vi "DB-通用exe查询模块.vi"(8 "error in (no error)":errorcluster, 9 "解析模式":enum16{"仅数值", "仅字符串", "数值与字符串", "不转换", "不抓取"}(ring)=enum."不抓取" caption="解析模式(不抓取)", 10 "SQL query":string, 11 "数据库连接引用":T1) -> (0 "error out":errorcluster, 1 "字符串数据":string[][](array[string]), 2 "数值数据":dbl[][](array[numeric]), 3 "数据库连接引用out":T1, 4 "recordset data":variant[][](array[variant]))   [LabVIEW 2017]
uses:
  <vilib>/addons/database/Connection.llb/Conn ObjectReference.ctl
  <vilib>/addons/database/Connection.llb/Conn Execute.vi
  <vilib>/addons/database/Recordset.llb/Rec Fetch Recordset Data (R).vi
  <vilib>/addons/database/Recordset.llb/Rec Destroy - Connection.vi
  <vilib>/addons/database/_DB Variant To Data/Database Variant To Data.xnode
  <vilib>/addons/database/NI_Database_API.lvlib
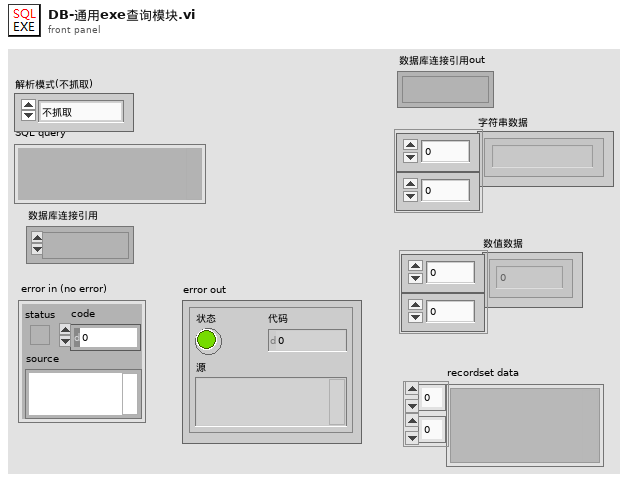
[diagram p1: front panel]
types:
  T1 = typedef "NI_Database_API.lvlib/Conn ObjectReference.ctl" = refnum<k1>
  T2 = typedef "NI_Database_API.lvlib/Rec ObjectReference.ctl" = refnum<k1>
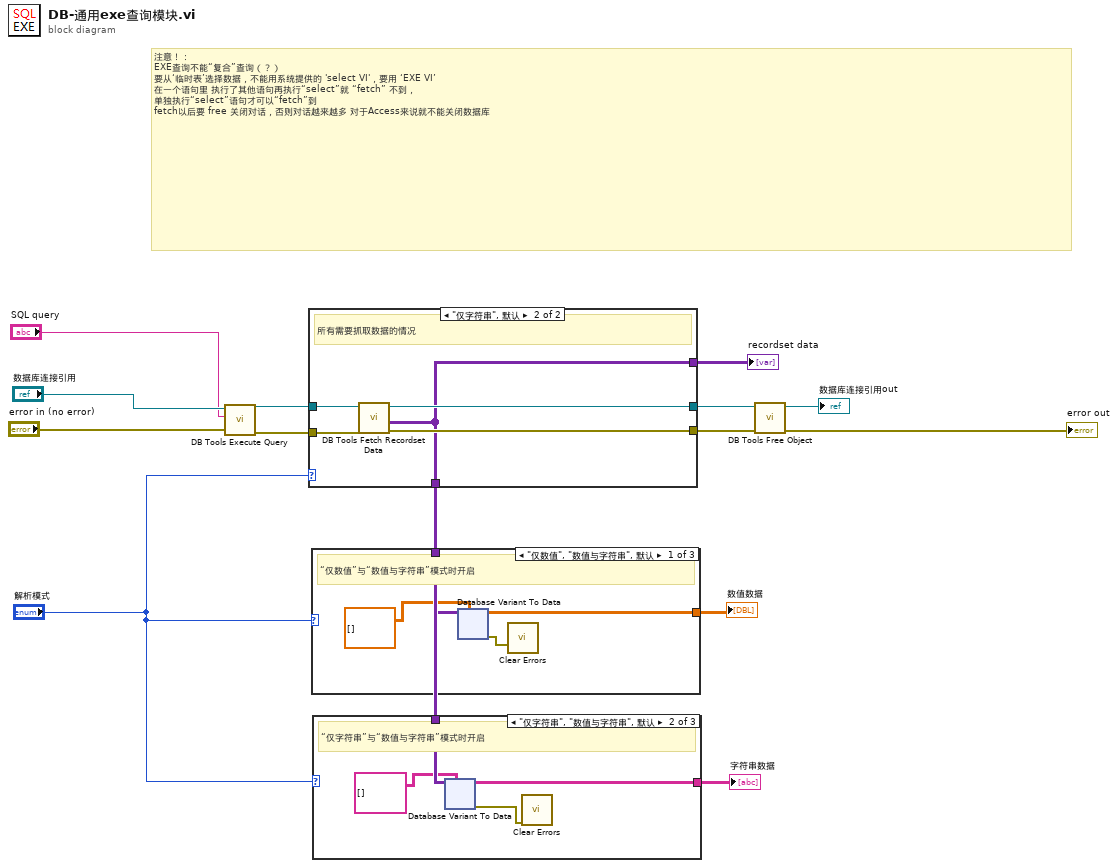
[diagram p0: block diagram]
diagram:
  # "注意！：\nEXE查询不能“复合”查询（？）\n要从‘临时表’选择数据，不能用系统提供的 'select VI'，要用 ‘EXE VI’\n在一个语句里 执行了其他语句再执行“select”就 “fetch” 不到，\n单独执行“select”语句才可以“fetch”到\nfetch以后要 free 关闭对话，否则对话越来越多 对于Access来说就不能关闭数据库"
  n1 = call-poly <vilib>:"DB Tools Execute Query.vi"("error in (no error)"="error in (no error)", "SQL query"="SQL query", "connection reference"="数据库连接引用") -> ("error out"=w13:errorcluster, "recordset reference"=w12:T2)  [unwired: 5 in]
  n2 = case shown="\"仅字符串\", 默认" "解析模式" {
    tunnel: w13 -> [w15 w21]
    tunnel: w12 -> [w16 w20]
    tunnel: [_ w17] -> w9
    tunnel: [w16 w19] -> w8
    tunnel: [w15 w18] -> w7
    tunnel: [_ w17] -> w1
    frame "不抓取" {
      # "不需要抓取的情况"
    }
    frame "仅字符串", Default {
      # "所有需要抓取数据的情况"
      n3 = call-poly <vilib>:"DB Tools Fetch Recordset Data.vi"("error in (no error)"=w21, "recordset reference"=w20) -> ("error out"=w18:errorcluster, "recordset data"=w17:variant[][], "recordset reference out"=w19:T2)  [unwired: 3 in]
    }
  }
  "recordset data" <- w1
  n4 = case shown="\"仅数值\", \"数值与字符串\", 默认" "解析模式" {
    tunnel: w9 -> [w24 _ _]
    tunnel: [w22 _ _] -> w3
    frame "仅数值", "数值与字符串", Default {
      # "“仅数值”与“数值与字符串”模式时开启"
      n5 = xnode "Database Variant To Data"("database variant"=w24, "type"=dbl[][] []) -> ("data"=w22:dbl[][], "error out"=w23:errorcluster)  [unwired: 1 in]
      n6 = call <vilib>:"Clear Errors.vi"("error in (no error)"=w23) -> ()  [unwired: 5 in, 2 out]
    }
    frame "仅字符串" {
    }
    frame "不转换" {
      # "不执行转换"
    }
  }
  "数值数据" <- w3
  n7 = case shown="\"仅字符串\", \"数值与字符串\", 默认" "解析模式" {
    tunnel: w9 -> [_ w73 _]
    tunnel: [_ w70 _] -> w2
    frame "仅数值" {
    }
    frame "仅字符串", "数值与字符串", Default {
      # "“仅字符串”与“数值与字符串”模式时开启"
      n8 = xnode "Database Variant To Data"("database variant"=w73, "type"=string[][] []) -> ("data"=w70:string[][], "error out"=w71:errorcluster)  [unwired: 1 in]
      n9 = call <vilib>:"Clear Errors.vi"("error in (no error)"=w71) -> ()  [unwired: 5 in, 2 out]
    }
    frame "不转换" {
      # "不执行转换"
    }
  }
  "字符串数据" <- w2
  n10 = call-poly <vilib>:"DB Tools Free Object.vi"("error in (no error)"=w7, "recordset reference"=w8) -> ("error out"=→"error out":errorcluster, "connection reference"=→"数据库连接引用out":T1)  [unwired: 8 in]
